vi "Configure High Volt Resistance.vi"(4 "Fast Conversion (F: OFF)":bool, 6 "Filter (F: OFF)":bool, 8 "error in (no error)":errorcluster, 9 "Connection (0:Two wire)":u16(ring) items=["Two wire", "Four wire"], 11 "VISA resource name":refnum<visa-resource-name>) -> (0 "error out":errorcluster, 3 "VISA resource name out":refnum<visa-resource-name>)   [LabVIEW 2012, in "Fluke 8508.lvlib"]
doc: "This VI sets High Voltage Resistance specific settings such as the connection, filtering and conversion type on the instrument.\n\nNOTE: This VI does not have to be run just to set the instrument to make High Voltage Resistance measurements, but instead it is meant to be a supplement to the \"Configure Measurement\" VI which sets the measurement function, range, and resolution."
uses:
  Fluke 8508.lvlib
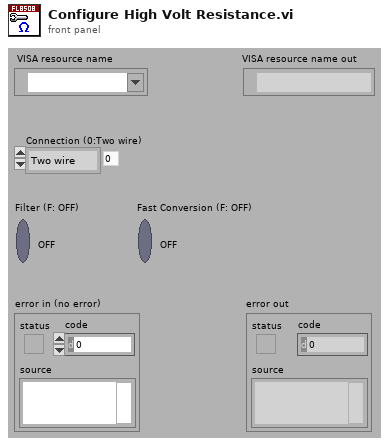
[diagram p1: front panel]
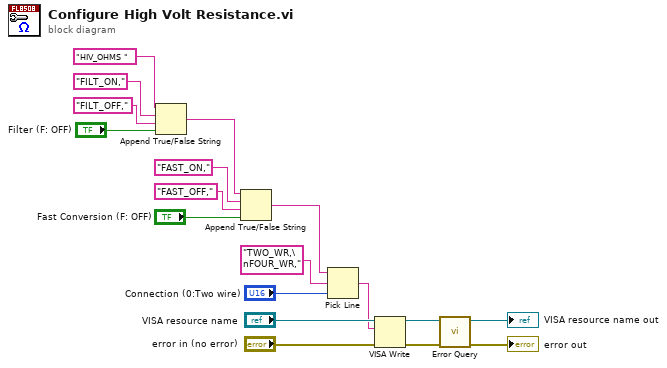
[diagram p0: block diagram]
diagram:
  n1 = Append True/False String(1:"Filter (F: OFF)", 2:"FILT_OFF," ("false string"), 3:"FILT_ON," ("true string"), 4:"HIV_OHMS ") -> (0:w5:string)
  n2 = Append True/False String(1:"Fast Conversion (F: OFF)", 2:"FAST_OFF," ("false string"), 3:"FAST_ON," ("true string"), 4:w5) -> (0:w10:string)
  n3 = Pick Line(string ("")=w10, multi-line string="TWO_WR,\nFOUR_WR," ("true string"), line index="Connection (0:Two wire)") -> (output string=w7:string)
  n4 = VISA Write(VISA resource name="VISA resource name", write buffer=w7, error in (no error)="error in (no error)") -> (VISA resource name out=w2:refnum<visa-resource-name>, error out=w4:errorcluster)  [unwired: 1 out]
  n5 = call "Error Query.vi"("error in (no error)"=w4, "VISA resource name"=w2) -> ("error out"=→"error out":errorcluster, "VISA resource name out"=→"VISA resource name out":refnum<visa-resource-name>)  [unwired: 6 in, 2 out]
